vi "ReadContinous.vi"(8 "error in (no error)":errorcluster, 9 "Max samples to keep":u32, 10 "Min samples to read":u32, 11 "Scope5761 in":refnum<class "Scope5761.lvclass">) -> (0 "error out":errorcluster, 1 "#elements":i32, 2 "Data":dbl[][](array[numeric]), 3 "Scope5761 out":refnum<class "Scope5761.lvclass">)   [LabVIEW 2013, in "Scope5761.lvclass"]
uses:
  Scope5761.lvclass
  Scope5761.lvclass/Scope5761.ctl
  FpgaRef/FpgaRef5761/FpgaRef5761.lvclass
  FpgaRef/FpgaRef5782/FpgaRef5782.lvclass
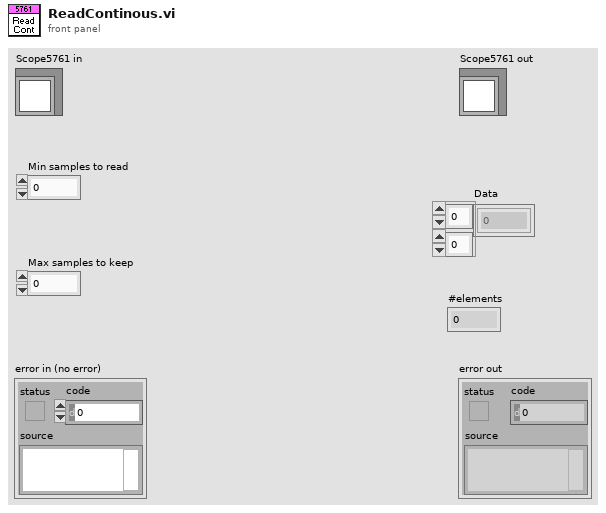
[diagram p1: front panel]
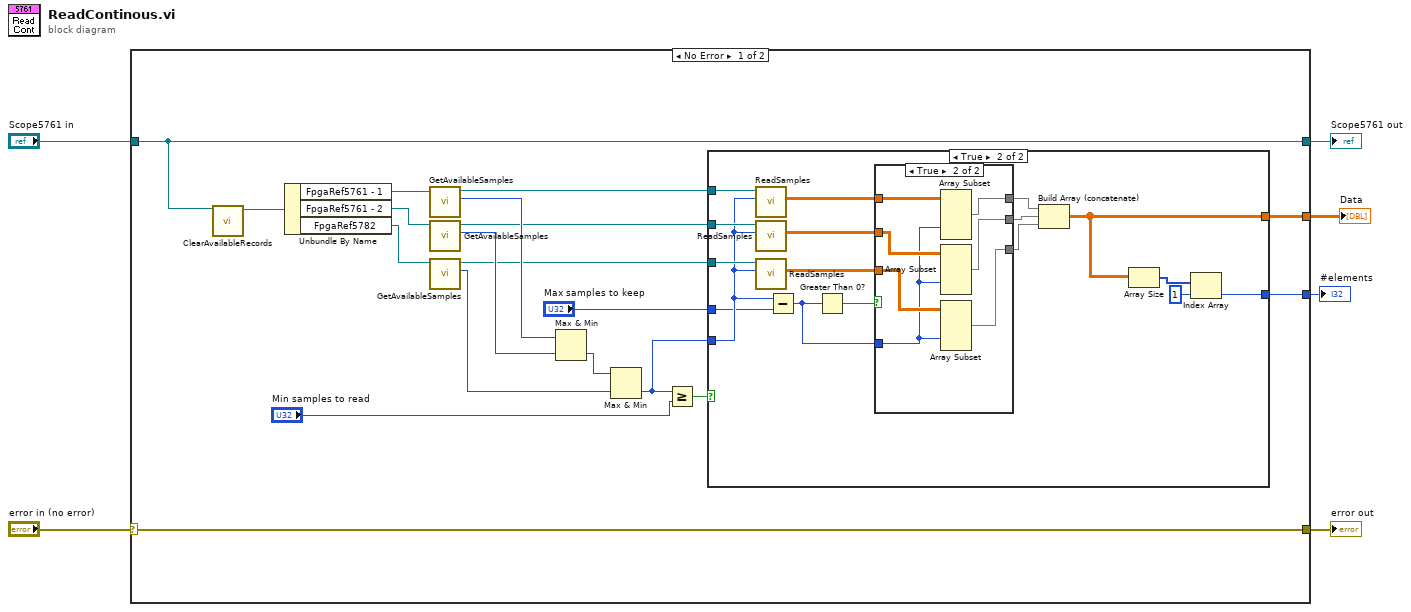
[diagram p0: block diagram]
diagram:
  n1 = case shown="No Error" "error in (no error)" {
    selector: "error in (no error)" -> [w25 w54]
    tunnel: [w25 w54] -> w5
    tunnel: [w22 w53] -> w3
    tunnel: "Scope5761 in" -> [w22 w53]
    tunnel: [w24 _] -> w2
    tunnel: [w23 _] -> w1
    frame No Error {
      n2 = call "ClearAvailableRecords.vi"("Scope5761 in"=w22) -> ("Scope5761 out"=w21:refnum<class "Scope5761.lvclass">)  [unwired: 9 in, 1 out]
      n3 = Unbundle By Name(w21) -> ("FpgaRef5761 - 1"=w20:refnum<class "FpgaRef5761.lvclass">, "FpgaRef5761 - 2"=w19:refnum<class "FpgaRef5761.lvclass">, "FpgaRef5782"=w18:refnum<class "FpgaRef5782.lvclass">)
      n4 = call-dynamic "GetAvailableSamples.vi"("FpgaRef5761 In"=w20) -> ("available"=w17:u32, "FpgaRef5761 Out"=w9:refnum<class "FpgaRef5761.lvclass">)  [unwired: 8 in, 1 out]
      n5 = call-dynamic "GetAvailableSamples.vi"("FpgaRef5761 In"=w19) -> ("available"=w16:u32, "FpgaRef5761 Out"=w8:refnum<class "FpgaRef5761.lvclass">)  [unwired: 8 in, 1 out]
      n6 = call-dynamic "GetAvailableSamples.vi"("FpgaRef5782 in"=w18) -> ("available"=w14:u32, "FpgaRef5782 out"=w7:refnum<class "FpgaRef5782.lvclass">)  [unwired: 8 in, 1 out]
      n7 = Max & Min(x=w17, y=w16) -> (min(x,y)=w15:u32)  [unwired: 1 out]
      n8 = Max & Min(x=w15, y=w14) -> (min(x,y)=w11:u32)  [unwired: 1 out]
      n9 = Greater Or Equal?(x=w11, y="Min samples to read") -> (x >= y?=w12:bool)
      n10 = case shown="True" w12 {
        tunnel: [_ w42] -> w24
        tunnel: [_ w39] -> w23
        tunnel: w11 -> [_ w34]
        tunnel: "Max samples to keep" -> [_ w33]
        tunnel: w9 -> [_ w38]
        tunnel: w8 -> [_ w37]
        tunnel: w7 -> [_ w36]
        frame False {
        }
        frame True {
          n11 = call-dynamic "ReadSamples.vi"("Num samples to read"=w34, "FpgaRef5761 In"=w38) -> ("Data"=w35:dbl[][])  [unwired: 7 in, 2 out]
          n12 = call-dynamic "ReadSamples.vi"("Num samples to read"=w34, "FpgaRef5761 In"=w37) -> ("Data"=w32:dbl[][])  [unwired: 7 in, 2 out]
          n13 = call-dynamic "ReadSamples.vi"("Num samples to read"=w34, "FpgaRef5782 in"=w36) -> ("Data"=w27:dbl[][])  [unwired: 7 in, 2 out]
          n14 = Subtract(x=w34, y=w33) -> (x-y=w31:u32)
          n15 = Greater Than 0?(x=w31) -> (x > 0?=w30:bool)
          n16 = case shown="True" w30 {
            tunnel: w35 -> [w45 w52]
            tunnel: w32 -> [w44 w50]
            tunnel: w31 -> [_ w46]
            tunnel: [w45 w51] -> w29
            tunnel: [w44 w49] -> w28
            tunnel: w27 -> [w43 w48]
            tunnel: [w43 w47] -> w26
            frame False {
            }
            frame True {
              n17 = Array Subset(array=w52, index (col)=w46) -> (w51:dbl[][])  [unwired: 3 in]
              n18 = Array Subset(array=w50, index (col)=w46) -> (w49:dbl[][])  [unwired: 3 in]
              n19 = Array Subset(array=w48, index (col)=w46) -> (w47:dbl[][])  [unwired: 3 in]
            }
          }
          n20 = Build Array (concatenate)(w29, w28, w26) -> (w42:dbl[][])
          n21 = Array Size(array=w42) -> (size(s)=w41:i32[])
          n22 = Index Array(array=w41, index=1) -> (element=w39:i32)
        }
      }
    }
    frame Error {
    }
  }
  "error out" <- w5
  "Scope5761 out" <- w3
  "Data" <- w2
  "#elements" <- w1
